vi "Global modalità avvio.vi"() -> ()   [LabVIEW 2016]
panel:
  in  "Modalità avvio":T1={"MODALITA' BANCO"=enum."BANCO FRENO", "MODALITA' AVVIO MOTORE"=enum."AVVIO A TENSIONE RIDOTTA", "MODALITA' AVVIO FRENO"=enum."MARCIA PRIMA AVVIO", "V avvio[V]"=0.0, "F avvio[Hz]"=0.0, "%V ridotta"=0.0, "C avvio [Nm]"=0.0, "RPM avvio"=0.0, "SERVO AVVIO"=FALSE}
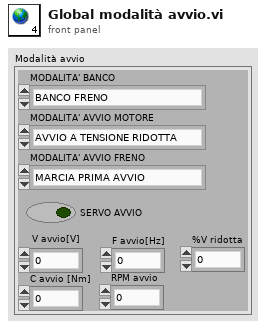
[diagram p1: front panel]
types:
  T1 = typedef "Modalità avvio.ctl" = cluster{"MODALITA' BANCO":enum32{"BANCO FRENO", "SOLO ALIMENTATORE", "SOLO TRASCINAMENTO", "GESTIONE MANUALE"}, "MODALITA' AVVIO MOTORE":enum32{"AVVIO A TENSIONE RIDOTTA", "AVVIO IN RAMPA", "AVVIO DIRETTO DA ALIM", "AVVIO DIRETTO DA LINEA"}, "MODALITA' AVVIO FRENO":enum32{"MARCIA DOPO AVVIO MOTORE", "MARCIA PRIMA AVVIO"}, "V avvio[V]":dbl, "F avvio[Hz]":dbl, "%V ridotta":dbl, "C avvio [Nm]":dbl, "RPM avvio":dbl, "SERVO AVVIO":bool}
diagram:
